vi "unused_Read bounds.vi"(8 "error in (no error)":errorcluster, 11 "GObject in":refnum<class "GObject.lvclass">) -> (0 "error out":errorcluster, 3 "GObject out":refnum<class "GObject.lvclass">)   [LabVIEW 2023]
uses:
  GObject.lvclass/GObject.ctl
  GObject.lvclass
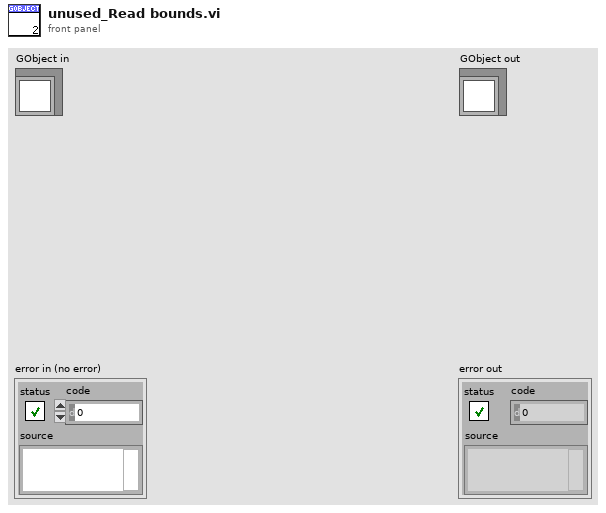
[diagram p1: front panel]
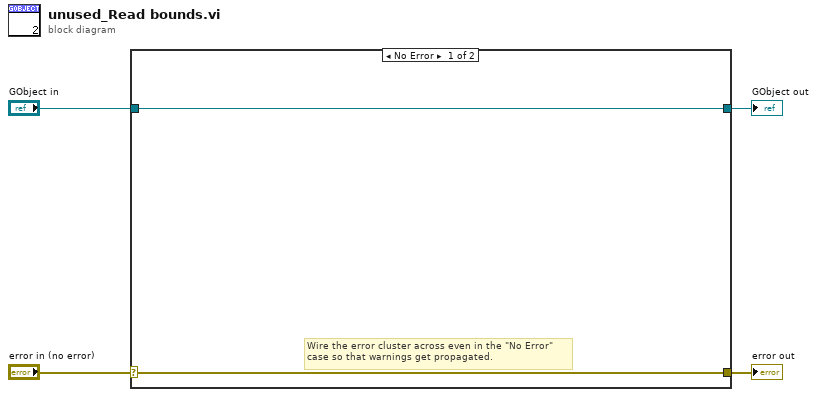
[diagram p0: block diagram]
diagram:
  n1 = case shown="No Error" "error in (no error)" {
    selector: "error in (no error)" -> [w5 w8]
    tunnel: [w5 w8] -> w3
    tunnel: [w6 w7] -> w1
    tunnel: "GObject in" -> [w6 w7]
    frame No Error {
      # "Wire the error cluster across even in the \"No Error\"\ncase so that warnings get propagated."
    }
    frame Error {
    }
  }
  "error out" <- w3
  "GObject out" <- w1
